vi "Action VI on Download.vi"(6 "IP address":string, 7 "Details Ref":refnum<vi>, 8 "error in (no error)":errorcluster, 10 "ftp session":T2, 11 "Device Item Ref in":T1 format="%.0x") -> (0 "error out":errorcluster, 2 "ftp session out":T2, 3 "Device Item Ref out":T1 format="%.0x")   [LabVIEW 2009, in "NI-XNET Custom Device.lvlib"]
doc: "This VI is automatically called when the channel configuration is downloaded to the RT target. Look at the .xml file to see how to enable this VI to be called automatically."
uses:
  NI-XNET Custom Device.lvlib
  <vilib>/addons/internet/ftp/ftp0.llb/FTP Session.ctl
  <vilib>/NI VeriStand/Custom Device API/Custom Device Item Ref.ctl
  <vilib>/NI VeriStand/Custom Device API/Get Item Property (Variant).vi
  <vilib>/NI VeriStand/Custom Device API/Custom Device API.lvlib
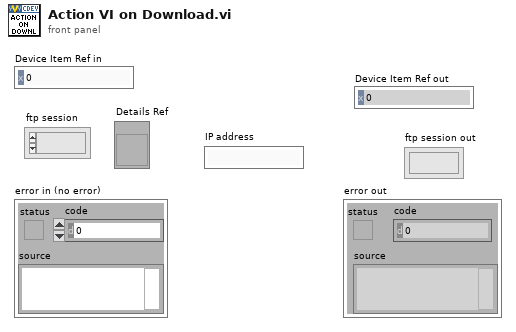
[diagram p1: front panel]
types:
  T1 = typedef "Custom Device API.lvlib/Custom Device Item Ref.ctl" = u64
  T2 = typedef "FTP Session.ctl" = refnum<k1>
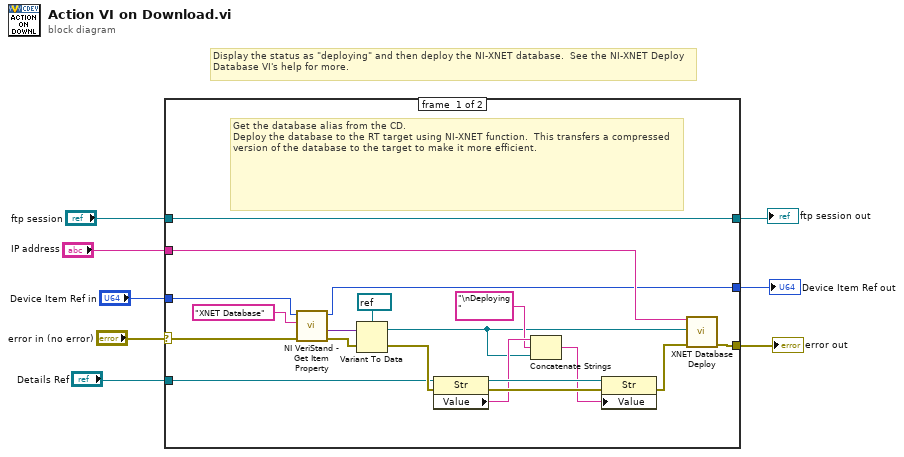
[diagram p0: block diagram]
diagram:
  # "Display the status as \"deploying\" and then deploy the NI-XNET database.  See the NI-XNET Deploy Database VI's help for more."
  n1 = case shown="No Error" "error in (no error)" {
    selector: "error in (no error)" -> [w24 w30]
    tunnel: [w26 w30] -> w7
    tunnel: "ftp session" -> [w18 w29]
    tunnel: [w18 w29] -> w5
    tunnel: "Device Item Ref in" -> [w25 w28]
    tunnel: [w19 w28] -> w3
    tunnel: "IP address" -> [w27 _]
    tunnel: "Details Ref" -> [w9 _]
    frame #0 {
      # "Get the database alias from the CD. \nDeploy the database to the RT target using NI-XNET function.  This transfers a compressed version of the database to the target to make it more efficient."
      n2 = call-poly <vilib>:"NI VeriStand - Get Item Property.vi"("error in (no error)"=w24, "Property Name"="XNET Database", "Item Ref in"=w25) -> ("error out"=w20:errorcluster, "Value"=w21:variant, "Item Ref out"=w19:T1)  [unwired: 5 in, 1 out]
      n3 = Variant To Data(error in=w20, Variant=w21, type=refnum<k21> refnum ("XNET Database 2")) -> (error out=w13:errorcluster, data=w10:refnum<k21>)
      n4 = property class="Str"(reference=w9, error in=w13) -> (reference out=w17:refnum<vi>, error out=w16:errorcluster, "Value"=w15:string)
      n5 = Concatenate Strings(w15, "\nDeploying " ("message"), w10) -> (w14:string)
      n6 = property class="Str"(reference=w17, error in=w16, "Value"=w14) -> (error out=w12:errorcluster)  [unwired: 1 out]
      n7 = call <vilib>:"XNET Database Deploy.vi"("IP address"=w27, "alias"=w10, "error in (no error)"=w12) -> ("error out"=w26:errorcluster)  [unwired: 11 in, 1 out]
    }
    frame #1 {
    }
  }
  "error out" <- w7
  "ftp session out" <- w5
  "Device Item Ref out" <- w3
